vi "Get XNET Signal Names.vi"(6 "Add Info?":bool, 7 "Parent Ref in":T1 format="%.0x", 8 "error in":errorcluster, 9 "Tree In":refnum<vi>, 10 "Parent":string, 11 "Frms":refnum<k21>[](array[refnum])) -> (0 "error out":errorcluster, 1 "Tree Out":refnum<vi>, 3 "XNET Signal Names":refnum<k21>[](array[refnum]))   [LabVIEW 2019, in "Protection and Counter Addon System Explorer.lvlib"]
uses:
  Protection and Counter Addon System Explorer.lvlib
  <vilib>/NI VeriStand/Custom Device API/Custom Device Item Ref.ctl
  <vilib>/NI VeriStand/Custom Device API/Custom Device Channel.ctl
  <vilib>/NI VeriStand/Custom Device API/Custom Device Channel Type.ctl
  Addon Shared/SubVIs/GUID Lookup.vi
  <vilib>/NI VeriStand/Custom Device API/Set Item Property (U32).vi
  <resource>/objmgr/xnet.rc
  <vilib>/NI VeriStand/Custom Device API/Custom Device API.lvlib
  Addon Shared/Protection and Counter Addon Shared.lvlib
  <vilib>/NI VeriStand/Custom Device Tools/Custom Device Utility Library/Custom Device Utility Library.lvlib
  <vilib>/NI VeriStand/Custom Device Tools/Custom Device Utility Library/NI VeriStand - Search for Item by Name.vi
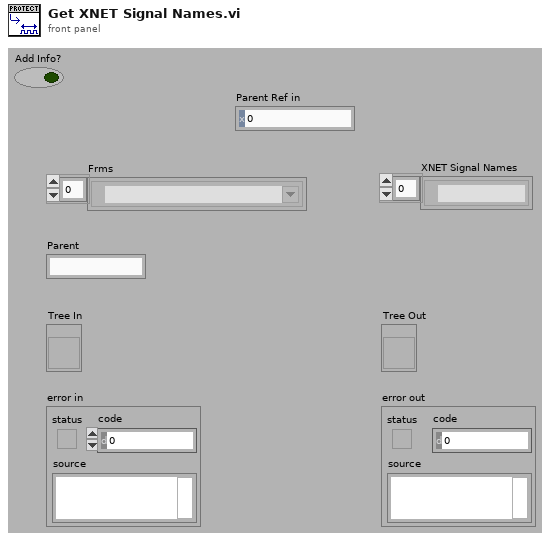
[diagram p1: front panel]
types:
  T1 = typedef "Custom Device API.lvlib/Custom Device Item Ref.ctl" = u64
  T2 = typedef "Custom Device API.lvlib/Custom Device Channel.ctl" = cluster{"Type":T3, "Units":string, "Default Value":dbl, "Faultable":bool, "Scalable":bool}
  T3 = typedef "Custom Device API.lvlib/Custom Device Channel Type.ctl" = enum16{"Input", "Output"}
  T4 = typedef "Custom Device API.lvlib/Custom Device Item Info.ctl" = cluster{"Name":string, "Is Channel":bool, "GUID":string, "Is Waveform":bool}
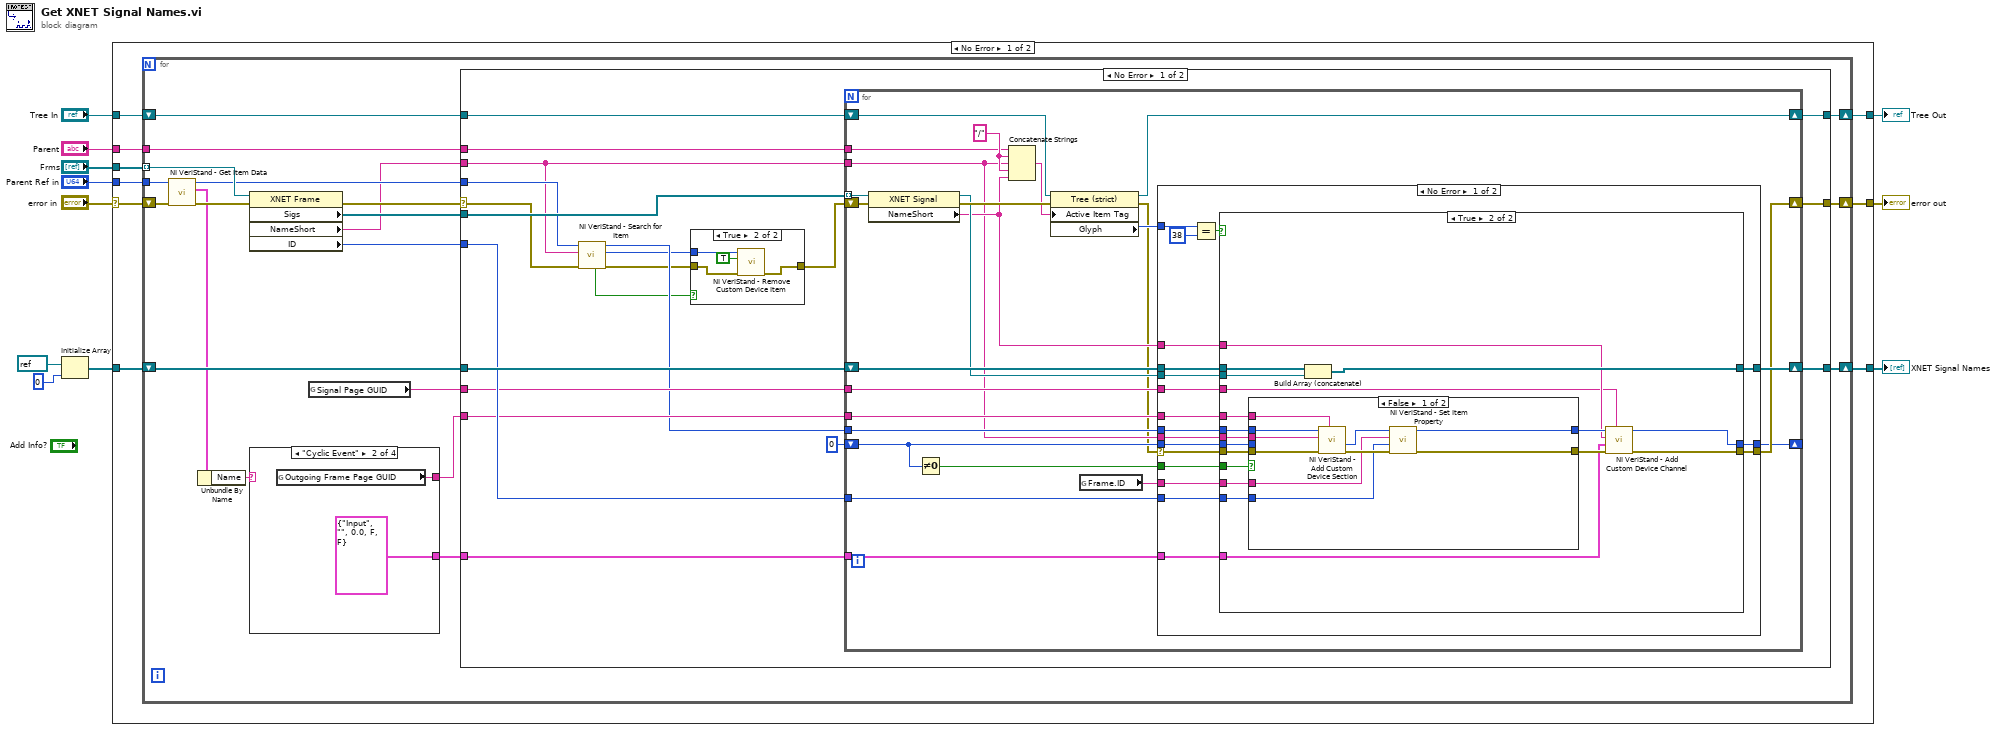
[diagram p0: block diagram]
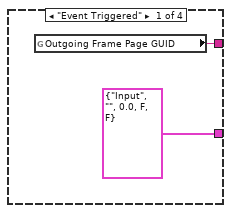
[diagram p2: hidden frame]
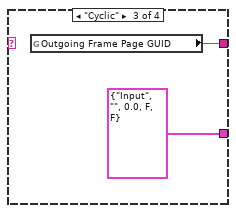
[diagram p3: hidden frame]
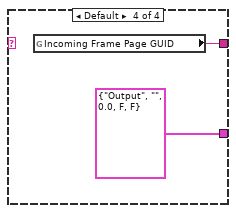
[diagram p4: hidden frame]
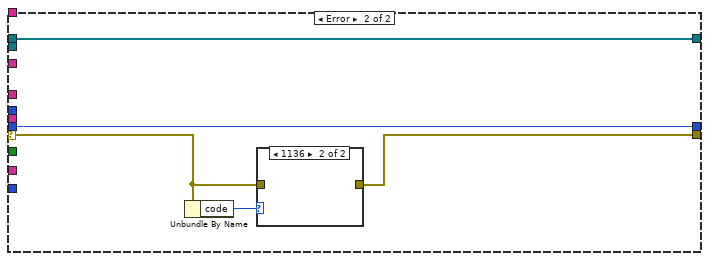
[diagram p8: hidden frame]
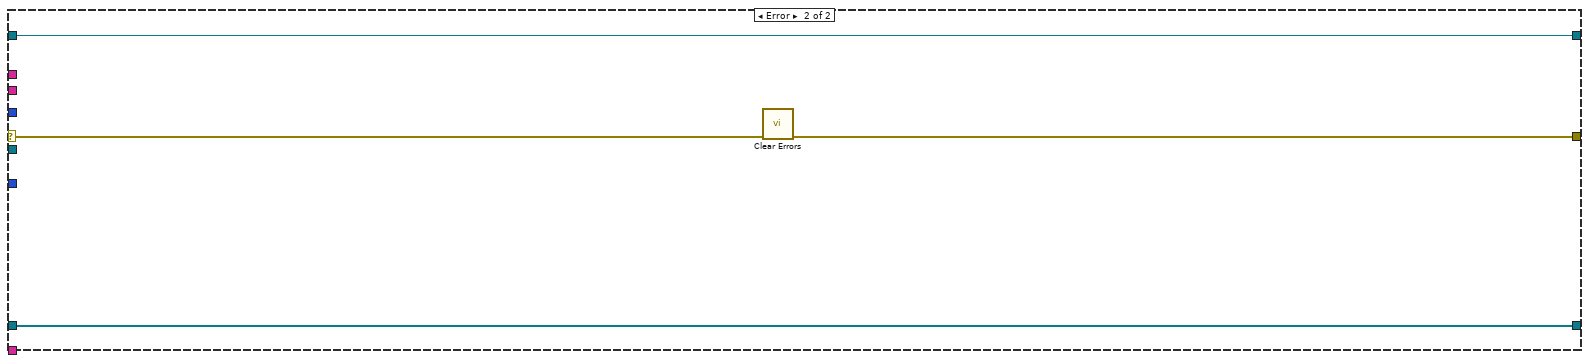
[diagram p10: hidden frame]
diagram:
  n1 = Initialize Array(refnum<k21> refnum ("XNET Signal"), 0 ("dimension size")) -> (w5:refnum<k21>[])
  n2 = case shown="No Error" "error in" {
    selector: "error in" -> [w17 w162]
    tunnel: "Parent" -> [w20 _]
    tunnel: [w19 w162] -> w10
    tunnel: "Frms" -> [w18 _]
    tunnel: [w16 _] -> w7
    tunnel: w5 -> [w15 _]
    tunnel: "Tree In" -> [w14 w161]
    tunnel: [w13 w161] -> w2
    tunnel: "Parent Ref in" -> [w12 _]
    frame No Error {
      n3 = for {
        shift-right: [w37] -> w19
        shift-left: w17 -> [w31]
        tunnel: w18 -> [w40] mode=indexing
        tunnel: w20 -> [w38]
        shift-right: [w34] -> w16
        shift-left: w15 -> [w35]
        shift-right: [w33] -> w13
        shift-left: w14 -> [w36]
        tunnel: w12 -> [w29]
        n4 = call <vilib>:"NI VeriStand - Get Item Data.vi"("error in (no error)"=w31, "Item Ref in"=w29) -> ("error out"=w30:errorcluster, "Item Info"=w27:T4, "Item Ref out"=w28:T1)  [unwired: 7 out]
        n5 = Unbundle By Name(w27) -> ("Name"=w26:string)
        n6 = property class="XNET Frame"(reference=w40, error in=w30) -> (error out=w32:errorcluster, "Sigs"=w39:refnum<k21>[], "NameShort"=w24:string, "ID"=w23:u32)  [unwired: 1 out]
        n7 = case shown="\"Cyclic Event\"" w26 {
          tunnel: [T2 {"Type"=enum."Input", "Units"="", "Default Value"=0.0, "Faultable"=FALSE, "Scalable"=FALSE} ("Channel") T2 {"Type"=enum."Input", "Units"="", "Default Value"=0.0, "Faultable"=FALSE, "Scalable"=FALSE} ("Channel") T2 {"Type"=enum."Input", "Units"="", "Default Value"=0.0, "Faultable"=FALSE, "Scalable"=FALSE} ("Channel") T2 {"Type"=enum."Output", "Units"="", "Default Value"=0.0, "Faultable"=FALSE, "Scalable"=FALSE} ("Channel")] -> w25
          tunnel: [w41 w43 w45 w47] -> w22
          frame "Event Triggered" {
            n8 = global read "GUID Lookup.vi" "Outgoing Frame Page GUID"() -> (w41:string)
          }
          frame "Cyclic Event" {
            n9 = global read "GUID Lookup.vi" "Outgoing Frame Page GUID"() -> (w43:string)
          }
          frame "Cyclic" {
            n10 = global read "GUID Lookup.vi" "Outgoing Frame Page GUID"() -> (w45:string)
          }
          frame Default {
            n11 = global read "GUID Lookup.vi" "Incoming Frame Page GUID"() -> (w47:string)
          }
        }
        n12 = global read "GUID Lookup.vi" "Signal Page GUID"() -> (w21:string)
        n13 = case shown="No Error" w32 {
          selector: w32 -> [w56 w157]
          tunnel: w39 -> [w68 _]
          tunnel: w24 -> [w53 _]
          tunnel: w38 -> [w67 _]
          tunnel: [w66 w158] -> w37
          tunnel: w36 -> [w65 w159]
          tunnel: w35 -> [w64 w160]
          tunnel: [w63 w160] -> w34
          tunnel: [w62 w159] -> w33
          tunnel: w28 -> [w54 _]
          tunnel: w23 -> [w60 _]
          tunnel: w21 -> [w59 _]
          tunnel: w22 -> [w58 _]
          tunnel: w25 -> [w57 _]
          frame No Error {
            n14 = call-poly <vilib>:"NI VeriStand - Search for Item.vi"("error in"=w56, "Item Name"=w53, "Section Ref in"=w54) -> ("error out"=w50:errorcluster, "Item Ref"=w51:T1, "Section Ref out"=w55:T1, "Found"=w52:bool)  [unwired: 5 in]
            n15 = case shown="True" w52 {
              tunnel: w51 -> [_ w73]
              tunnel: w50 -> [w69 w72]
              tunnel: [w69 w71] -> w49
              frame False {
              }
              frame True {
                n16 = call <vilib>:"NI VeriStand - Remove Custom Device Item.vi"("error in (no error)"=w72, "Force Delete (F)"=TRUE, "Item Ref in"=w73) -> ("error out"=w71:errorcluster)  [unwired: 7 in, 1 out]
              }
            }
            n17 = for {
              tunnel: w68 -> [w98] mode=indexing
              tunnel: w53 -> [w76]
              tunnel: w67 -> [w95]
              shift-right: [w86] -> w66
              shift-left: w49 -> [w97]
              shift-right: [w90] -> w63
              shift-left: w64 -> [w89]
              shift-right: [w87] -> w62
              shift-left: w65 -> [w93]
              tunnel: w55 -> [w85]
              shift-right: [w84] -> _
              shift-left: T1 0 ("Parent Ref out") -> [w83]
              tunnel: w60 -> [w80]
              tunnel: w59 -> [w79]
              tunnel: w58 -> [w78]
              tunnel: w57 -> [w77]
              w96 = "/" ("string")
              n18 = property class="XNET Signal"(reference=w98, error in=w97) -> (reference out=w88:refnum<k21>, error out=w94:errorcluster, "NameShort"=w81:string)
              n19 = Not Equal To 0?(x=w83) -> (x != 0?=w82:bool)
              n20 = Concatenate Strings(w95, w96, w76, w96, w81) -> (w92:string)
              n21 = property class="Tree (strict)"(reference=w93, error in=w94, "Active Item Tag"=w92) -> (reference out=w87:refnum<vi>, error out=w75:errorcluster, "Glyph"=w91:i32)
              n22 = global read "GUID Lookup.vi" "Frame.ID"() -> (w74:string)
              n23 = case shown="No Error" w75 {
                selector: w75 -> [w99 w152]
                tunnel: w91 -> [w117 _]
                tunnel: [w114 w154] -> w90
                tunnel: w89 -> [w113 w154]
                tunnel: w88 -> [w112 _]
                tunnel: [w111 w151] -> w86
                tunnel: w85 -> [w110 _]
                tunnel: [w109 w155] -> w84
                tunnel: w83 -> [w108 w155]
                tunnel: w82 -> [w107 _]
                tunnel: w81 -> [w106 _]
                tunnel: w80 -> [w105 _]
                tunnel: w74 -> [w104 _]
                tunnel: w79 -> [w103 _]
                tunnel: w78 -> [w102 _]
                tunnel: w77 -> [w101 _]
                tunnel: w76 -> [w100 _]
                frame No Error {
                  n24 = Equal?(x=w117, y=38) -> (x = y?=w115:bool)
                  n25 = case shown="True" w115 {
                    tunnel: [w120 w136] -> w114
                    tunnel: w113 -> [w120 w138]
                    tunnel: w112 -> [_ w137]
                    tunnel: w107 -> [_ w135]
                    tunnel: w100 -> [_ w134]
                    tunnel: w99 -> [w119 w133]
                    tunnel: [w119 w121] -> w111
                    tunnel: w110 -> [_ w132]
                    tunnel: [w118 w129] -> w109
                    tunnel: w108 -> [w118 w131]
                    tunnel: w106 -> [_ w127]
                    tunnel: w102 -> [_ w126]
                    tunnel: w103 -> [_ w125]
                    tunnel: w105 -> [_ w124]
                    tunnel: w104 -> [_ w123]
                    tunnel: w101 -> [_ w122]
                    frame False {
                    }
                    frame True {
                      n26 = case shown="False" w135 {
                        tunnel: w134 -> [w148 _]
                        tunnel: w133 -> [w147 w150]
                        tunnel: [w140 w150] -> w130
                        tunnel: w132 -> [w146 _]
                        tunnel: [w139 w149] -> w128
                        tunnel: w131 -> [_ w149]
                        tunnel: w126 -> [w145 _]
                        tunnel: w124 -> [w141 _]
                        tunnel: w123 -> [w142 _]
                        frame False {
                          n27 = call <vilib>:"NI VeriStand - Add Custom Device Section.vi"("GUID (Default Section)"=w145, "error in (no error)"=w147, "Section Name"=w148, "Parent Ref in"=w146) -> ("error out"=w143:errorcluster, "Section Ptr"=w144:T1)  [unwired: 4 in, 2 out]
                          n28 = call-poly <vilib>:"NI VeriStand - Set Item Property.vi"("error in (no error)"=w143, "Value"=w141, "Property Name"=w142, "Item Ref in"=w144) -> ("error out"=w140:errorcluster, "Item Ref out"=w139:T1)  [unwired: 5 in, 1 out]
                        }
                        frame True {
                        }
                      }
                      n29 = Build Array (concatenate)(w138, w137) -> (w136:refnum<k21>[])
                      n30 = call <vilib>:"NI VeriStand - Add Custom Device Channel.vi"("GUID (Default Channel)"=w125, "error in (no error)"=w130, "Channel"=w122, "Channel Name"=w127, "Parent Ref in"=w128) -> ("error out"=w121:errorcluster, "Parent Ref out"=w129:T1)  [unwired: 3 in, 2 out]
                    }
                  }
                }
                frame Error {
                  n31 = Unbundle By Name(w152) -> ("code"=w153:i32)
                  n32 = case shown="1136" w153 {
                    tunnel: [w156 _] -> w151
                    tunnel: w152 -> [w156 _]
                    frame Default {
                    }
                    frame 1136 {
                    }
                  }
                }
              }
            }
          }
          frame Error {
            n33 = call <vilib>:"Clear Errors.vi"("error in (no error)"=w157) -> ("error out"=w158:errorcluster)  [unwired: 5 in, 1 out]
          }
        }
      }
    }
    frame Error {
    }
  }
  "error out" <- w10
  "XNET Signal Names" <- w7
  "Tree Out" <- w2
